vi "macro_NumCmd_Send_OneDbl.vi"() -> ()   [LabVIEW 2019, in "Trajectory_Library.lvlib"]
uses:
  VI/numCmd_ObtainQueue_OneDbl.vi
  Trajectory_Library.lvlib
panel:
  in  "ElevatorHeightDemand-Ft":dbl
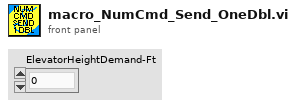
[diagram p1: front panel]
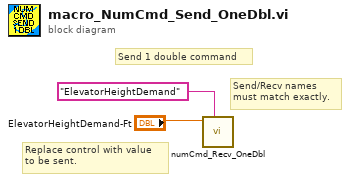
[diagram p0: block diagram]
diagram:
  # "Send/Recv names\nmust match exactly."
  # "Replace control with value \nto be sent."
  # "Send 1 double command"
  n1 = call "numCmd_Recv_OneDbl.vi"("Command Name"="ElevatorHeightDemand", "Initial Value"="ElevatorHeightDemand-Ft") -> ()  [unwired: 7 in, 3 out]
